vi "Write Numeric Scalar to Source (Base16 I16).vi"(8 "width (4)":i16=4, 9 "offset":i32, 10 "value":i16, 11 "error in":errorcluster) -> (1 "new offset":i32, 3 "error out":errorcluster)   [LabVIEW 2020, in "Static Errors.lvlib"]
doc: "Converts <b>value</b> into an hexadecimal-formatted string, and writes the string to the <b>error in</b> source buffer at the specified <b>offset</b>."
uses:
  Static Errors.lvlib
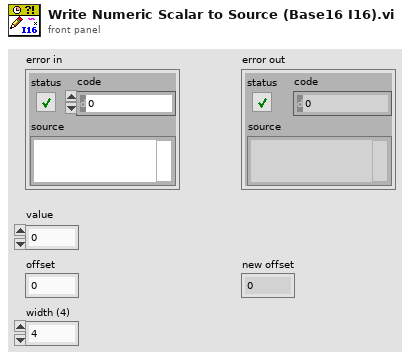
[diagram p1: front panel]
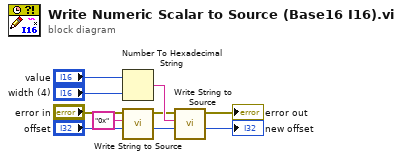
[diagram p0: block diagram]
diagram:
  n1 = Number To Hexadecimal String(1:"width (4)", 2:"value") -> (0:w8:string)
  n2 = call "Write String to Source.vi"("offset"="offset", "string"="0x", "error in"="error in") -> ("new offset"=w4:i32, "error out"=w5:errorcluster)  [unwired: 7 in]
  n3 = call "Write String to Source.vi"("offset"=w4, "string"=w8, "error in"=w5) -> ("new offset"=→"new offset":i32, "error out"=→"error out":errorcluster)  [unwired: 7 in]
